vi "Status LED.vi"() -> ()   [LabVIEW 2020, in "CTI-Scratchpad.lvlib"]
uses:
  CTI-Scratchpad.lvlib
  CTI/Status Source.ctl
  CTI/ADC Number.ctl
  CTI/Session/Session.lvclass
  CTI/VisaComms/VisaComms.lvclass
  CTI/CTI.lvlib
panel:
  in  "User Status":bool
  in  "Speed":i32(slide)=101 scale=1000.0..1.0
  in  "stop":bool
  in  "Port":refnum<visa-resource-name>="COM3"
  out "Current Source":T1
  out "ADC":u16(graph)
  in  "User Source":bool
  in  "Comms Source":bool
  # "Set Source:"
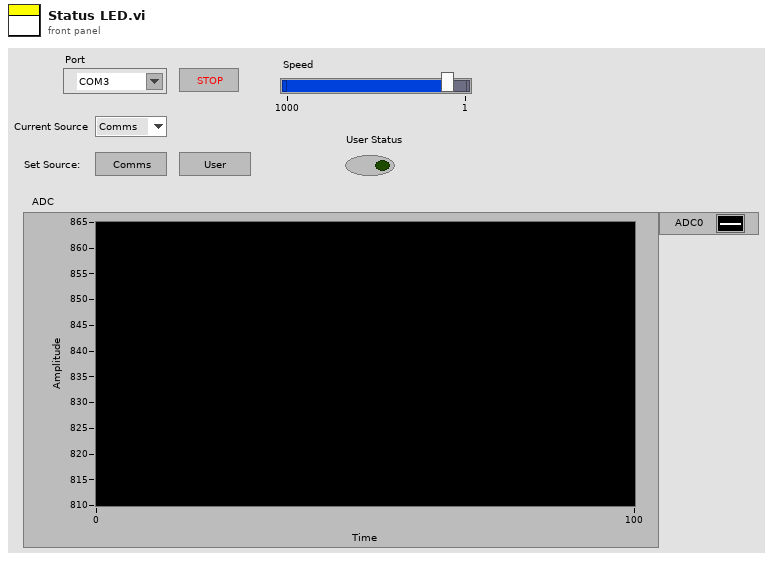
[diagram p1: front panel]
types:
  T1 = typedef "CTI.lvlib/Status Source.ctl" = enum16{"Comms", "User"}
  T2 = typedef "CTI.lvlib/ADC Number.ctl" = i8
  T3 = typedef "CTI.lvlib/Raw ADC.ctl" = u16
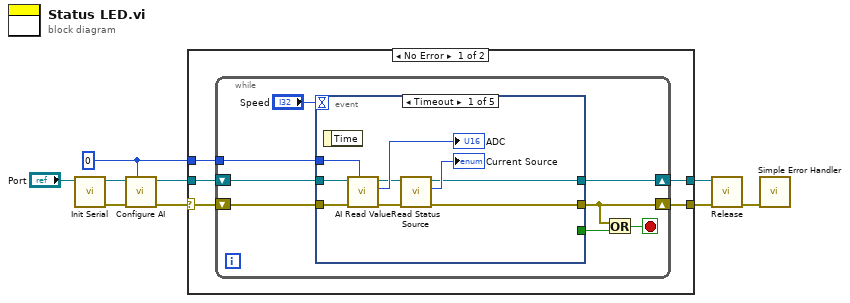
[diagram p0: block diagram]
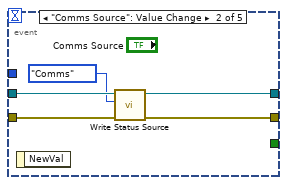
[diagram p2: hidden frame]
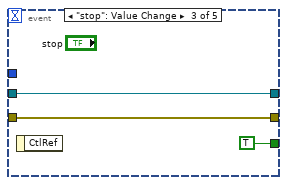
[diagram p3: hidden frame]
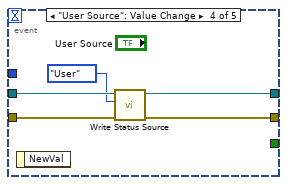
[diagram p4: hidden frame]
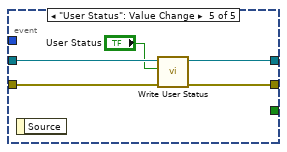
[diagram p5: hidden frame]
diagram:
  w1 = T2 0 ("Channel")
  n1 = call "Init Serial.vi"("VISA resource name in"="Port") -> ("error out"=w7:errorcluster, "Session"=w8:refnum<class "Session.lvclass">)  [unwired: 8 in, 1 out]
  n2 = call "Configure AI.vi"("ADC #"=w1, "error in (no error)"=w7, "Session in"=w8) -> ("error out"=w6:errorcluster, "Session out"=w5:refnum<class "Session.lvclass">)  [unwired: 7 in]
  n3 = case shown="No Error" w6 {
    selector: w6 -> [w13 w50]
    tunnel: w5 -> [w14 w51]
    tunnel: w1 -> [w12 _]
    tunnel: [w11 w51] -> w3
    tunnel: [w10 w50] -> w2
    frame No Error {
      n4 = while {
        shift-right: [w17] -> w10
        shift-left: w13 -> [w20]
        shift-right: [w18] -> w11
        shift-left: w14 -> [w21]
        tunnel: w12 -> [w19]
        stop <- w16 stop-if-true
        n5 = event shown="[0] Timeout" {
          selector: _ -> [_ _ _ _ _]
          dyn-events: _ -> [_ _ _ _ _]
          timeout: "Speed" -> [_ _ _ _ _]
          tunnel: w21 -> [w31 w36 w39 w44 w49]
          tunnel: w20 -> [w30 w35 w38 w43 w48]
          tunnel: w19 -> [w23 _ _ _ _]
          tunnel: [w25 w33 w39 w41 w46] -> w18
          tunnel: [w24 w32 w38 w40 w47] -> w17
          tunnel: [_ _ TRUE _ _] -> w15
          event Timeout {
            n6 = event-data() -> ()  [unwired: 1 in, 1 out]
            n7 = call "AI Read Value.vi"("ADC #"=w23, "error in (no error)"=w30, "Session in"=w31) -> ("error out"=w27:errorcluster, "Value"=→"ADC":T3, "Session out"=w28:refnum<class "Session.lvclass">)  [unwired: 6 in]
            n8 = call "Read Status Source.vi"("error in (no error)"=w27, "Session in"=w28) -> ("error out"=w24:errorcluster, "Status Source"=→"Current Source":T1, "Session out"=w25:refnum<class "Session.lvclass">)  [unwired: 7 in]
          }
          event "Comms Source": Value Change {
            n9 = event-data() -> ()  [unwired: 1 in, 1 out]
            n10 = call "Write Status Source.vi"("error in (no error)"=w35, "Status Source"=Status_Source."Comms", "Session in"=w36) -> ("error out"=w32:errorcluster, "Session out"=w33:refnum<class "Session.lvclass">)  [unwired: 7 in]
          }
          event "stop": Value Change {
            n11 = event-data() -> ()  [unwired: 1 in, 1 out]
          }
          event "User Source": Value Change {
            n12 = event-data() -> ()  [unwired: 1 in, 1 out]
            n13 = call "Write Status Source.vi"("error in (no error)"=w43, "Status Source"=Status_Source."User", "Session in"=w44) -> ("error out"=w40:errorcluster, "Session out"=w41:refnum<class "Session.lvclass">)  [unwired: 7 in]
          }
          event "User Status": Value Change {
            n14 = event-data() -> ()  [unwired: 1 in, 1 out]
            n15 = call "Write User Status.vi"("error in (no error)"=w48, "User Status"="User Status", "Session in"=w49) -> ("error out"=w47:errorcluster, "Session out"=w46:refnum<class "Session.lvclass">)  [unwired: 7 in]
          }
        }
        n16 = Or(x=w17, y=w15) -> (x .or. y?=w16:bool)
      }
    }
    frame Error {
    }
  }
  n17 = call-dynamic "Release.vi"("error in (no error)"=w2, "Session in"=w3) -> ("error out"=w4:errorcluster)  [unwired: 9 in]
  n18 = call <vilib>:"Simple Error Handler.vi"("error in (no error)"=w4) -> ()  [unwired: 4 in, 5 out]
